vi "acc_test.vi"(10 "Sample Rate":dbl, 11 "Data":dbl[][](array[numeric])) -> ()   [LabVIEW 2016]
uses:
  <vilib>/Analysis/NI_AALPro.lvlib
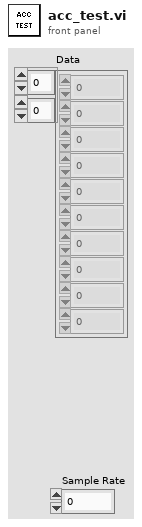
[diagram p1: front panel]
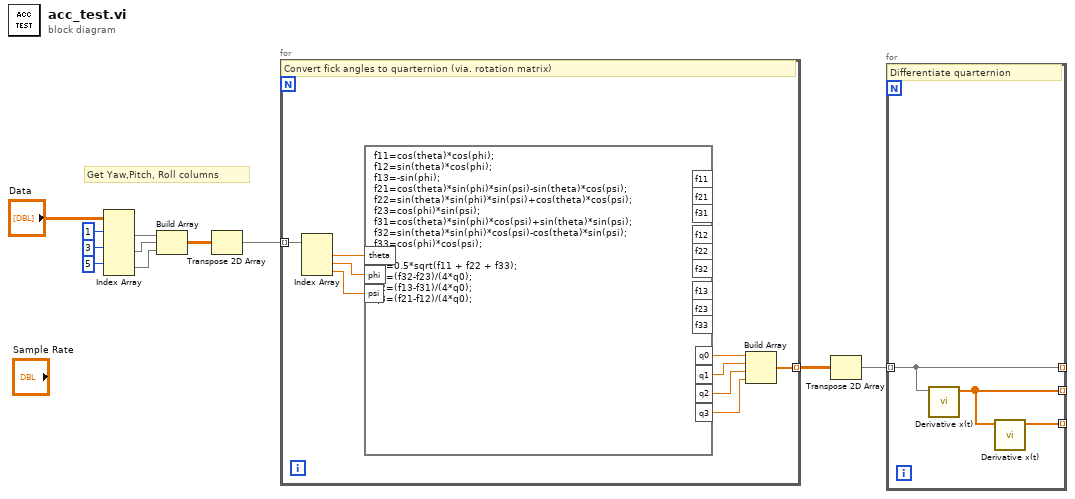
[diagram p0: block diagram]
diagram:
  # "Get Yaw,Pitch, Roll columns"
  n1 = Index Array(array="Data", index (row) #1=1 ("index (row)"), index (row) #2=3 ("index (row)"), index (row) #3=5 ("index (row)")) -> (element #1=w7:dbl[], element #2=w6:dbl[], element #3=w5:dbl[])  [unwired: 3 in]
  n2 = Build Array(w7, w6, w5) -> (w4:dbl[][])
  n3 = Transpose 2D Array(2D array=w4) -> (transposed array=w3:dbl[][])
  n4 = for {
    tunnel: w3 -> [w20] mode=indexing
    tunnel: [w12] -> w2 mode=indexing
    # "Convert fick angles to quarternion (via. rotation matrix)"
    n5 = Index Array(array=w20) -> (element #1=w19:dbl, element #2=w18:dbl, element #3=w17:dbl)  [unwired: 3 in]
    n6 = formula code="f11=cos(theta)*cos(phi);\nf12=sin(theta)*cos(phi);\nf13=-sin(phi);\nf21=cos(theta)*sin(phi)*sin(psi)-sin(theta)*cos(psi);\nf22=sin(theta)*sin(phi)*sin(psi)+cos(theta)*cos(psi);\nf23=cos(phi)*sin(psi);\nf31=cos(theta)*sin(phi)*cos(psi)+sin(theta)*sin(psi);\nf32=sin(theta)*sin(phi)*cos(psi)-cos(theta)*sin(psi);\nf33=cos(phi)*cos(psi);\n\nq0=0.5*sqrt(f11 + f22 + f33);\nq1=(f32-f23)/(4*q0);\nq2=(f13-f31)/(4*q0);\nq3=(f21-f12)/(4*q0);"("theta"=w19, "phi"=w18, "psi"=w17) -> ("q0"=w16:dbl, "q1"=w15:dbl, "q2"=w14:dbl, "q3"=w13:dbl)  [unwired: 9 out]
    n7 = Build Array(w16, w15, w14, w13) -> (w12:dbl[])
  }
  n8 = Transpose 2D Array(2D array=w2) -> (transposed array=w1:dbl[][])
  n9 = for {
    tunnel: w1 -> [w23] mode=indexing
    tunnel: [w23] -> _ mode=indexing
    tunnel: [w22] -> _ mode=indexing
    tunnel: [w21] -> _ mode=indexing
    # "Differentiate quarternion"
    n10 = call <vilib>:"Derivative x(t).vi"("X"=w23) -> ("dX/dt"=w22:dbl[])  [unwired: 9 in, 1 out]
    n11 = call <vilib>:"Derivative x(t).vi"("X"=w22) -> ("dX/dt"=w21:dbl[])  [unwired: 9 in, 1 out]
  }
